vi "Send Final Positions.vi"(8 "error in (no error)":errorcluster, 9 "end test?":bool, 10 "switch queue":refnum<queue>, 11 "servo queue":refnum<queue>) -> (0 "error out":errorcluster)   [LabVIEW 2020]
uses:
  Hardware/Actuators/Servos/Servo.lvclass
  Hardware/General Hardware.lvclass
  Hardware/Actuators/Switches/Switch.lvclass
  C:/Users/jharw/Documents/1 Folder to Rule them All/UMD/Inflation-Apparatus/src/Hardware/Actuators/Actuator.lvclass
  C:/Users/jharw/Documents/1 Folder to Rule them All/UMD/Inflation-Apparatus/src/Hardware/General Hardware.lvclass
  C:/Users/jharw/Documents/1 Folder to Rule them All/UMD/Inflation-Apparatus/src/Hardware/Actuators/Servos/Servo.lvclass
  C:/Users/jharw/Documents/1 Folder to Rule them All/UMD/Inflation-Apparatus/src/Hardware/Actuators/Switches/Switch.lvclass
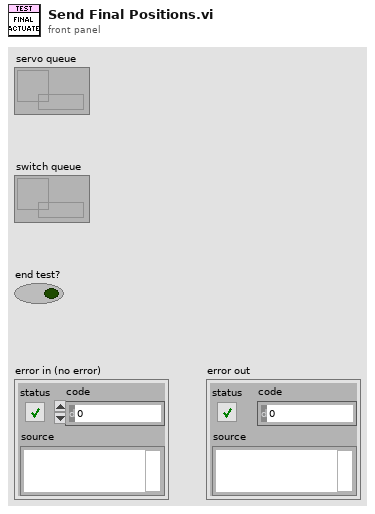
[diagram p1: front panel]
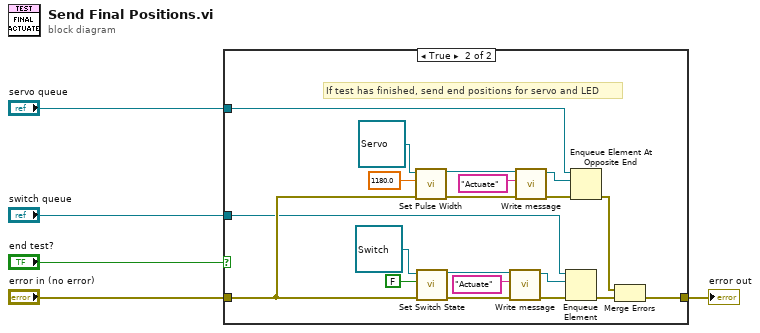
[diagram p0: block diagram]
diagram:
  n1 = case shown="True" "end test?" {
    tunnel: "error in (no error)" -> [w6 w11]
    tunnel: [w6 w9] -> w2
    tunnel: "servo queue" -> [_ w19]
    tunnel: "switch queue" -> [_ w7]
    frame False {
      # "Do nothing if test has not finished"
    }
    frame True {
      # "If test has finished, send end positions for servo and LED"
      n2 = call "Set Pulse Width.vi"("error in (no error)"=w11, "pulse width (micro-sec)"=1180.0, "Servo in"=refnum<class "Servo.lvclass"> refnum) -> ("error out"=w24:errorcluster, "Servo out"=w21:refnum<class "Servo.lvclass">)  [unwired: 7 in]
      n3 = call "Set Switch State.vi"("error in (no error)"=w11, "switch state"=FALSE, "Switch in"=refnum<class "Switch.lvclass"> refnum) -> ("error out"=w16:errorcluster, "Switch out"=w14:refnum<class "Switch.lvclass">)  [unwired: 7 in]
      n4 = call "Write message.vi"("error in (no error)"=w16, "message"="Actuate", "General Hardware in"=w14) -> ("error out"=w15:errorcluster, "General Hardware out"=w13:refnum<class "Switch.lvclass">)  [unwired: 7 in]
      n5 = call "Write message.vi"("error in (no error)"=w24, "message"="Actuate", "General Hardware in"=w21) -> ("error out"=w23:errorcluster, "General Hardware out"=w22:refnum<class "Servo.lvclass">)  [unwired: 7 in]
      n6 = Enqueue Element(queue=w7, element=w13, error in (no error)=w15) -> (error out=w10:errorcluster)  [unwired: 1 in, 2 out]
      n7 = Enqueue Element At Opposite End(queue=w19, element=w22, error in (no error)=w23) -> (error out=w8:errorcluster)  [unwired: 1 in, 2 out]
      n8 = Merge Errors(w8, w10) -> (w9:errorcluster)
    }
  }
  "error out" <- w2
